vi "create message.vi"(9 "response queue":refnum<queue>, 10 "data":variant, 11 "ID":string) -> (3 "message":refnum<class "communicator message.lvclass">)   [LabVIEW 2015, in "communicator message.lvclass"]
uses:
  communicator message.lvclass
  communicator message.lvclass/communicator message.ctl
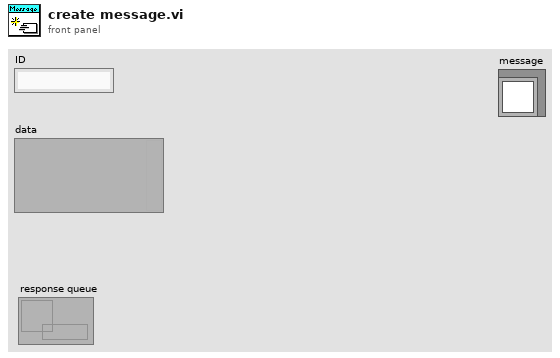
[diagram p1: front panel]
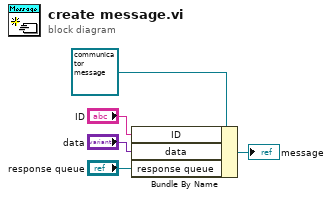
[diagram p0: block diagram]
diagram:
  n1 = Bundle By Name(cluster=refnum<class "communicator message.lvclass"> refnum ("message"), "ID"="ID", "data"="data", "response queue"="response queue") -> (→"message":refnum<class "communicator message.lvclass">)
